vi "FilterNextStates.vi"(7 "StateName":string, 8 "error in (no error)":errorcluster, 9 "QueueUsed(This means that the wire is connected to incoming queue elements)":bool, 10 "NextStates":T1[](array[typedef]), 11 "StateReverse in":refnum<class "StateReverse.lvclass">) -> (0 "error out":errorcluster, 1 "AlreadyAnalysed":bool=TRUE, 2 "NextStatesOut":T1[](array[typedef]), 3 "StateReverse out":refnum<class "StateReverse.lvclass">)   [LabVIEW 2020, in "StateReverse.lvclass"]
uses:
  <resource>/Framework/Providers/Open_GDS/UML/StateReverse_class/StateReverse.lvclass
  <resource>/Framework/Providers/Open_GDS/UML/StateReverse_class/NextStateAction.ctl
  <resource>/Framework/Providers/Open_GDS/UML/StateReverse_class/StateAction.ctl
  <resource>/Framework/Providers/Open_GDS/UML/StateReverse_class/StateReverse.lvclass/StateReverse.ctl
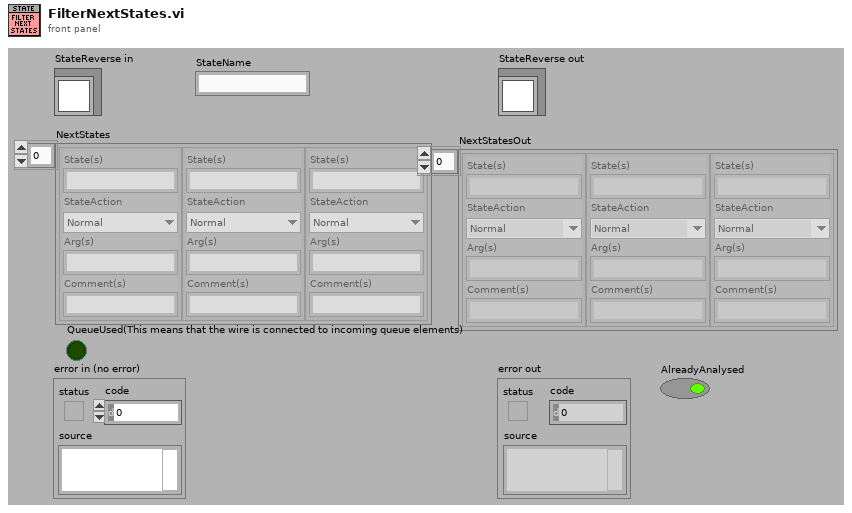
[diagram p1: front panel]
types:
  T1 = typedef "StateReverse.lvclass/NextStateAction.ctl" = cluster{"State(s)":string, "StateAction":T2, "Arg(s)":string, "Comment(s)":string}
  T2 = typedef "StateReverse.lvclass/StateAction.ctl" = enum16{"Normal", "AddInBeggining", "AddInEnd", "AddIfNothingInQueue"}
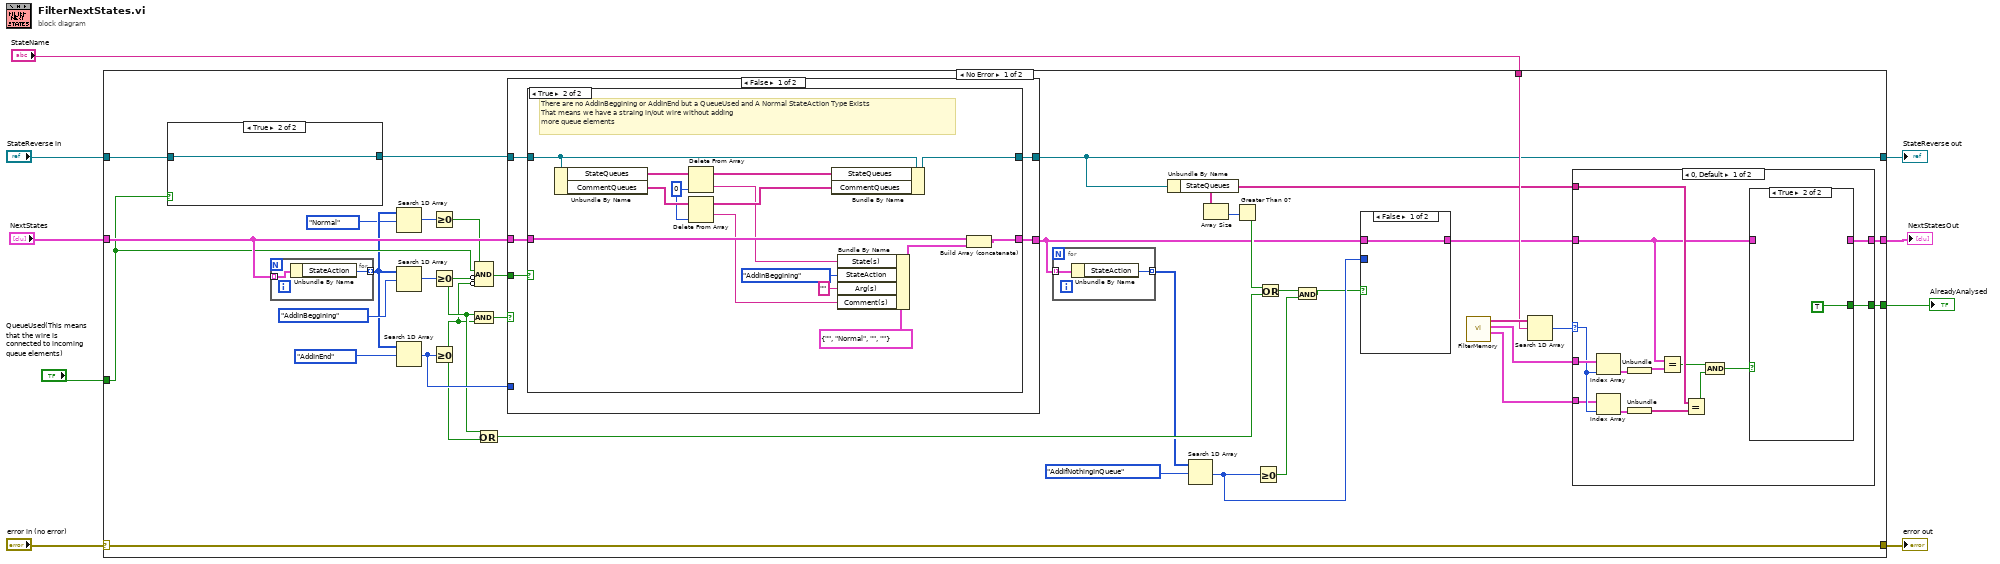
[diagram p0: block diagram]
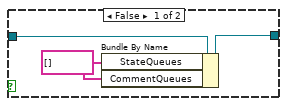
[diagram p4: hidden frame]
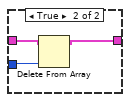
[diagram p5: hidden frame]
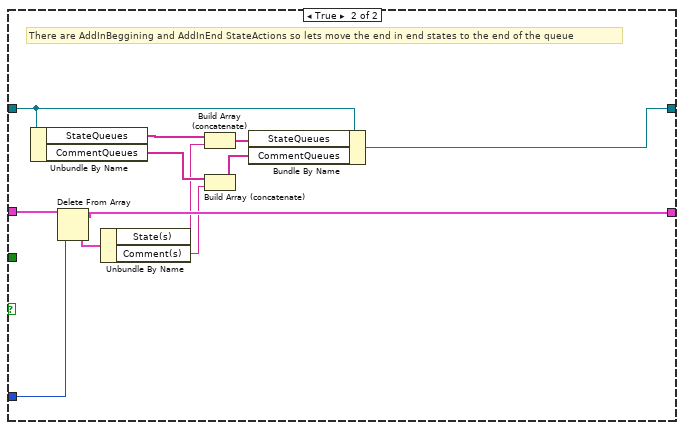
[diagram p7: hidden frame]
diagram:
  n1 = case shown="No Error" "error in (no error)" {
    selector: "error in (no error)" -> [w46 w112]
    tunnel: [w46 w112] -> w8
    tunnel: [w19 w111] -> w6
    tunnel: "StateReverse in" -> [w29 w111]
    tunnel: "NextStates" -> [w41 w110]
    tunnel: [w23 w110] -> w4
    tunnel: "QueueUsed(This means that the wire is connected to incoming queue elements)" -> [w16 _]
    tunnel: "StateName" -> [w26 _]
    tunnel: [w10 _] -> w1
    frame No Error {
      n2 = case shown="True" w16 {
        tunnel: w29 -> [w66 w67]
        tunnel: [w65 w67] -> w28
        frame False {
          w64 = string[] [] ("StateQueues")
          n3 = Bundle By Name(cluster=w66, "StateQueues"=w64, "CommentQueues"=w64) -> (w65:refnum<class "StateReverse.lvclass">)
        }
        frame True {
        }
      }
      n4 = for {
        tunnel: w41 -> [w109] mode=indexing
        tunnel: [w108] -> w14 mode=indexing
        n5 = Unbundle By Name(w109) -> ("StateAction"=w108:T2)
      }
      n6 = Search 1D Array(1D array=w14, element=StateAction."Normal") -> (index of element=w12:i32)  [unwired: 1 in]
      n7 = Search 1D Array(1D array=w14, element=StateAction."AddInBeggining") -> (index of element=w43:i32)  [unwired: 1 in]
      n8 = Search 1D Array(1D array=w14, element=StateAction."AddInEnd") -> (index of element=w40:i32)  [unwired: 1 in]
      n9 = Greater Or Equal To 0?(x=w12) -> (x >= 0?=w11:bool)
      n10 = Greater Or Equal To 0?(x=w43) -> (x >= 0?=w18:bool)
      n11 = Greater Or Equal To 0?(x=w40) -> (x >= 0?=w17:bool)
      n12 = And(x=w18, y=w17) -> (x .and. y?=w42:bool)
      n13 = Compound Arithmetic op=AND(w11, w16, invert w18, invert w17) -> (w15:bool)
      n14 = Or(x=w18, y=w17) -> (x .or. y?=w37:bool)
      n15 = case shown="False" w42 {
        tunnel: w41 -> [w75 w107]
        tunnel: w40 -> [_ w106]
        tunnel: [w74 w105] -> w31
        tunnel: w28 -> [w77 w99]
        tunnel: [w76 w96] -> w19
        tunnel: w15 -> [w78 _]
        frame False {
          n16 = case shown="True" w78 {
            tunnel: w77 -> [w80 w91]
            tunnel: [w80 w90] -> w76
            tunnel: w75 -> [w79 w95]
            tunnel: [w79 w94] -> w74
            frame False {
            }
            frame True {
              w87 = 0 ("index")
              # "There are no AddInBeggining or AddInEnd but a QueueUsed and A Normal StateAction Type Exists\nThat means we have a straing in/out wire without adding\nmore queue elements"
              n17 = Unbundle By Name(w91) -> ("StateQueues"=w93:string[], "CommentQueues"=w89:string[])
              n18 = Delete From Array(array=w93, index=w87) -> (deleted portion=w85:string, array with subset deleted=w92:string[])  [unwired: 1 in]
              n19 = Delete From Array(array=w89, index=w87) -> (deleted portion=w84:string, array with subset deleted=w88:string[])  [unwired: 1 in]
              n20 = Bundle By Name(cluster=w91, "StateQueues"=w92, "CommentQueues"=w88) -> (w90:refnum<class "StateReverse.lvclass">)
              n21 = Bundle By Name(cluster=T1 {"State(s)"="", "StateAction"=enum."Normal", "Arg(s)"="", "Comment(s)"=""} ("Cluster"), "State(s)"=w85, "StateAction"=StateAction."AddInBeggining", "Arg(s)"="", "Comment(s)"=w84) -> (w81:T1)
              n22 = Build Array (concatenate)(w95, w81) -> (w94:T1[])
            }
          }
        }
        frame True {
          # "There are AddInBeggining and AddInEnd StateActions so lets move the end in end states to the end of the queue"
          n23 = Unbundle By Name(w99) -> ("StateQueues"=w104:string[], "CommentQueues"=w103:string[])
          n24 = Delete From Array(array=w107, index=w106) -> (deleted portion=w102:T1, array with subset deleted=w105:T1[])  [unwired: 1 in]
          n25 = Unbundle By Name(w102) -> ("State(s)"=w101:string, "Comment(s)"=w100:string)
          n26 = Build Array (concatenate)(w104, w101) -> (w98:string[])
          n27 = Build Array (concatenate)(w103, w100) -> (w97:string[])
          n28 = Bundle By Name(cluster=w99, "StateQueues"=w98, "CommentQueues"=w97) -> (w96:refnum<class "StateReverse.lvclass">)
        }
      }
      n29 = for {
        tunnel: w31 -> [w69] mode=indexing
        tunnel: [w68] -> w30 mode=indexing
        n30 = Unbundle By Name(w69) -> ("StateAction"=w68:T2)
      }
      n31 = Unbundle By Name(w19) -> ("StateQueues"=w20:string[])
      n32 = Search 1D Array(1D array=w30, element=StateAction."AddIfNothingInQueue") -> (index of element=w33:i32)  [unwired: 1 in]
      n33 = Array Size(array=w20) -> (size(s)=w39:i32)
      n34 = Greater Than 0?(x=w39) -> (x > 0?=w38:bool)
      n35 = Greater Or Equal To 0?(x=w33) -> (x >= 0?=w34:bool)
      n36 = Or(x=w38, y=w37) -> (x .or. y?=w35:bool)
      n37 = And(x=w35, y=w34) -> (x .and. y?=w32:bool)
      n38 = case shown="False" w32 {
        tunnel: w31 -> [w70 w73]
        tunnel: [w70 w72] -> w24
        tunnel: w33 -> [_ w71]
        frame False {
        }
        frame True {
          n39 = Delete From Array(array=w73, index=w71) -> (array with subset deleted=w72:T1[])  [unwired: 1 in, 1 out]
        }
      }
      n40 = call <resource>:"FilterMemory.vi"() -> ("StateQueuesOut"=w21:cluster{"StateQueuesOut":string[]}[], "NextStates"=w22:cluster{"NextStates":T1[]}[], "StatesOut"=w27:string[])  [unwired: 8 in, 1 out]
      n41 = Search 1D Array(1D array=w27, element=w26) -> (index of element=w25:i32)  [unwired: 1 in]
      n42 = case shown="0, Default" w25 {
        selector: w25 -> [w57 _]
        tunnel: w24 -> [w48 w63]
        tunnel: [w49 w63] -> w23
        tunnel: w22 -> [w60 _]
        tunnel: w21 -> [w56 _]
        tunnel: w20 -> [w53 _]
        tunnel: [w47 _] -> w10
        frame 0, Default {
          n43 = Index Array(array=w60, index=w57) -> (element=w59:cluster{"NextStates":T1[]})
          n44 = Index Array(array=w56, index=w57) -> (element=w58:cluster{"StateQueuesOut":string[]})
          n45 = Unbundle(w59) -> ("NextStates"=w55:T1[])
          n46 = Unbundle(w58) -> ("StateQueuesOut"=w54:string[])
          n47 = Equal?(x=w48, y=w55) -> (x = y?=w52:bool)
          n48 = Equal?(x=w53, y=w54) -> (x = y?=w51:bool)
          n49 = And(x=w52, y=w51) -> (x .and. y?=w50:bool)
          n50 = case shown="True" w50 {
            tunnel: [w61 _] -> w49
            tunnel: w48 -> [w61 _]
            tunnel: [_ TRUE] -> w47
            frame False {
            }
            frame True {
            }
          }
        }
        frame -1 {
        }
      }
    }
    frame Error {
    }
  }
  "error out" <- w8
  "StateReverse out" <- w6
  "NextStatesOut" <- w4
  "AlreadyAnalysed" <- w1
